vi "acq.EL.vi"(5 "Delay":u16, 6 "mode":T1, 7 "DVR":T3, 8 "error in":errorcluster, 9 "# Acq in":i32, 10 "image":refnum<queue>) -> (0 "error out":errorcluster, 2 "Image Out":T2)   [LabVIEW 2020]
uses:
  6ca06af8-5255-4aa7-8013-97f442914d80.vi
  camera/camera.lvclass
  _controls/data.ref.ctl
  _controls/data.ctl
  _controls/state.ctl
  _controls/data.vars.ctl
  _controls/flip.ctl
  <vilib>/vision/Image Controls.llb/IMAQ Image.ctl
  _controls/mode.ctl
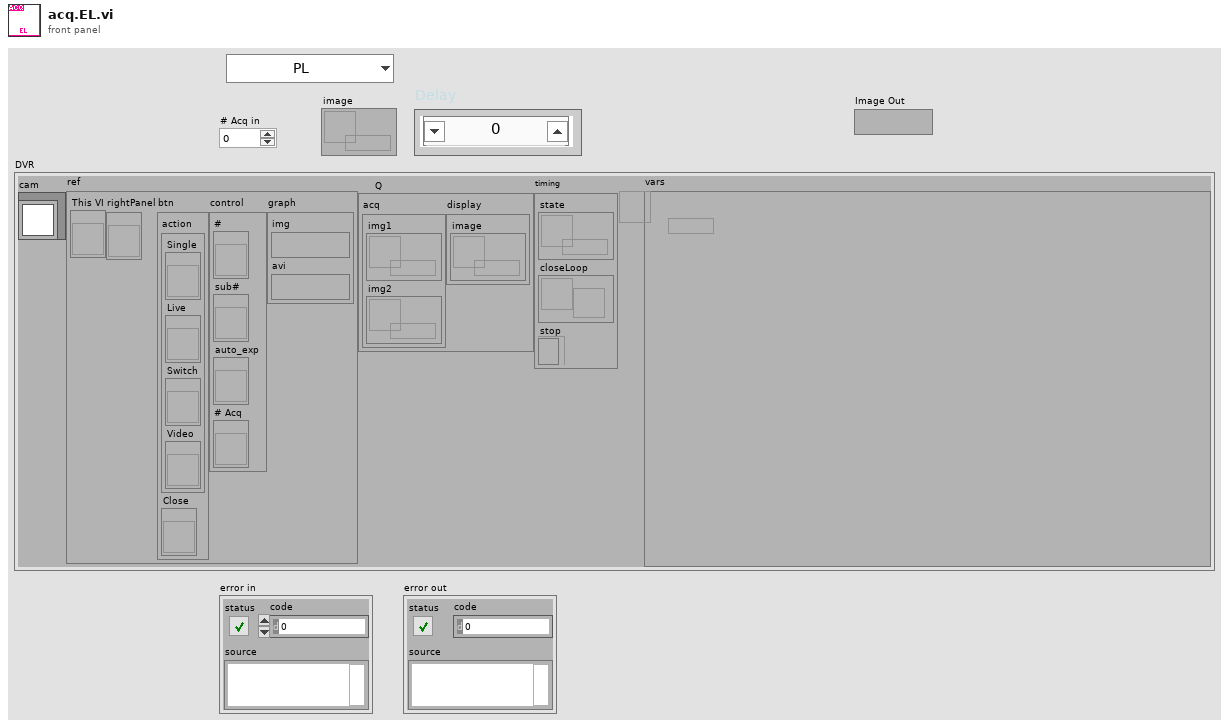
[diagram p1: front panel]
types:
  T1 = typedef "mode.ctl" = enum16{"PL", "EL"}
  T2 = typedef "IMAQ Image.ctl" = refnum<image>
  T3 = typedef "data.ctl" = cluster{"cam":refnum<class "camera.lvclass">, "ref":T4, "Q":cluster{"acq":cluster{"img1":refnum<queue>, "img2":refnum<queue>}, "display":cluster{"image":refnum<queue>}}, "timing":cluster{"state":refnum<queue>, "closeLoop":refnum<notifier>, "stop":refnum<k4>}, "vars":refnum<data-value>}
  T4 = typedef "data.ref.ctl" = cluster{"This VI":refnum<vi>, "rightPanel":refnum<vi>, "btn":cluster{"action":cluster{"Single":refnum<vi>, "Live":refnum<vi>, "Switch":refnum<vi>, "Video":refnum<vi>}, "Close":refnum<vi>}, "control":cluster{"#":refnum<vi>, "sub#":refnum<vi>, "auto_exp":refnum<vi>, "# Acq":refnum<vi>}, "graph":cluster{"img":T2, "avi":T2}}
  T5 = cluster{"img1":refnum<queue>, "img2":refnum<queue>}
  T6 = typedef "path.ctl" = cluster{"light":path, "name":string, "full":path}
  T7 = typedef "data.vars.ctl" = cluster{"save":cluster{"base_folder":cluster{"Folder":path, "tif":bool, "jpg":bool}, "module":string, "#":u32, "sub#":u8, "save.op":enum16{"Full", "Light"}, "same?":bool, "Shift":enum16{"Single", "Leapfrog"}, "jpg?":bool, "flip":T8}, "acq":cluster{"# Acq":u16, "rotate":bool, "FPS":dbl}, "calib.manual":cluster{"BG":cluster{"Image":u16[][], "enabled?":bool}, "FF":cluster{"Image":u16[][], "enabled?":bool}}}
  T8 = typedef "flip.ctl" = cluster{"x":bool, "y":bool}
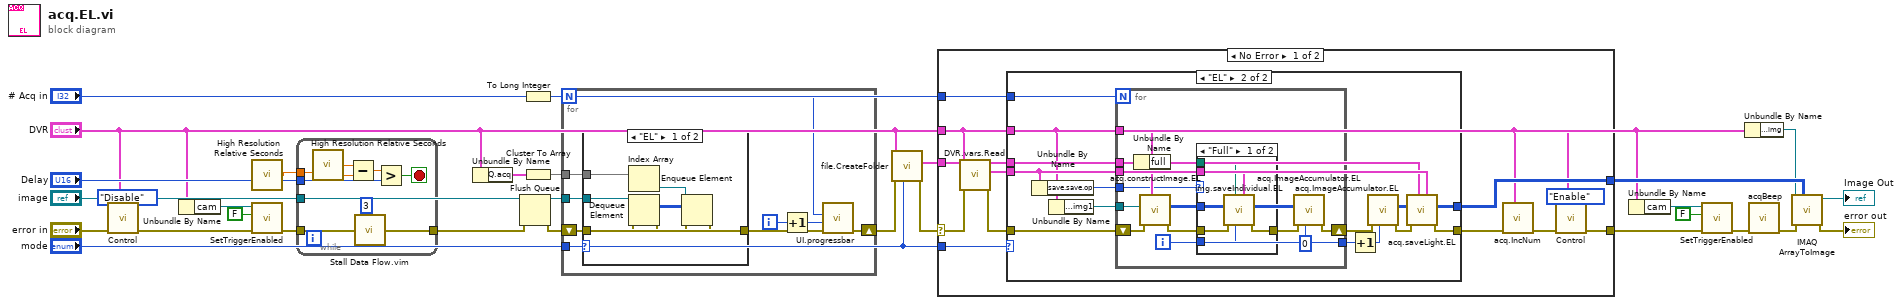
[diagram p0: block diagram]
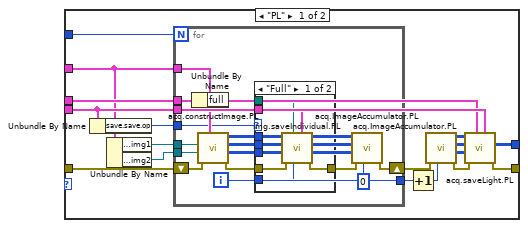
[diagram p2: hidden frame]
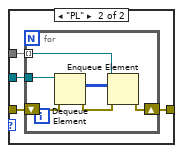
[diagram p6: hidden frame]
diagram:
  n1 = call "Control.vi"("mode"=enum16{"Enable", "Disable"}."Disable", "DVR"="DVR", "error in"="error in") -> ("error out"=w13:errorcluster)  [unwired: 8 in]
  n2 = Unbundle By Name("DVR") -> ("cam"=w14:refnum<class "camera.lvclass">)
  n3 = call <vilib>:"High Resolution Relative Seconds.vi"() -> ("relative seconds"=w18:dbl)
  n4 = call "SetTriggerEnabled.vi"("error in"=w13, "trigger"=FALSE, "camera.nit in"=w14) -> ("error out"=w12:errorcluster)  [unwired: 8 in]
  n5 = while {
    tunnel: "image" -> [_]
    tunnel: w18 -> [w36]
    tunnel: "Delay" -> [w34]
    tunnel: [w31] -> w5
    tunnel: w12 -> [w32]
    stop <- w33 stop-if-true
    n6 = call <vilib>:"High Resolution Relative Seconds.vi"() -> ("relative seconds"=w37:dbl)
    n7 = Subtract(x=w37, y=w36) -> (x-y=w35:dbl)
    n8 = call "Stall Data Flow.vim"("value in"=w32, "milliseconds to wait"=u32 3) -> ("value out"=w31:errorcluster)  [unwired: 1 out]
    n9 = Greater?(x=w35, y=w34) -> (0:w33:bool)
  }
  n10 = Unbundle By Name("DVR") -> ("Q.acq"=w23:T5)
  n11 = Flush Queue(queue="image", error in (no error)=w5) -> (queue out=w6:refnum<queue>, error out=w4:errorcluster)  [unwired: 1 out]
  n12 = To Long Integer(number="# Acq in") -> (32bit integer=w20:i32)
  n13 = Cluster To Array(cluster=w23) -> (array=w22:refnum<queue>[])
  n14 = for {
    N: w20 -> [w41]
    tunnel: w22 -> [w46]
    tunnel: w6 -> [w44]
    shift-right: [w40] -> _
    shift-left: w4 -> [w45]
    tunnel: "mode" -> [w38]
    i -> [w42]
    n15 = case shown="\"EL\"" w38 {
      tunnel: w46 -> [w53 w57]
      tunnel: w45 -> [w52 w56]
      tunnel: w44 -> [w51 w55]
      tunnel: [w50 w54] -> w43
      frame "EL" {
        n16 = Index Array(array=w53) -> (element=w47:refnum<queue>)  [unwired: 1 in]
        n17 = Dequeue Element(queue=w51, error in (no error)=w52) -> (element=w49:u16[][], error out=w48:errorcluster)  [unwired: 1 in, 2 out]
        n18 = Enqueue Element(queue=w47, element=w49, error in (no error)=w48) -> (error out=w50:errorcluster)  [unwired: 1 in, 2 out]
      }
      frame "PL" {
        n19 = for {
          tunnel: w55 -> [w63]
          tunnel: w57 -> [w62] mode=indexing
          shift-right: [w59] -> w54
          shift-left: w56 -> [w58]
          n20 = Dequeue Element(queue=w63, error in (no error)=w58) -> (element=w61:u16[][], error out=w60:errorcluster)  [unwired: 1 in, 2 out]
          n21 = Enqueue Element(queue=w62, element=w61, error in (no error)=w60) -> (error out=w59:errorcluster)  [unwired: 1 in, 2 out]
        }
      }
    }
    n22 = Increment(x=w42) -> (x+1=w39:i32)
    n23 = call "UI.progressbar.vi"("error in"=w43, "Value"=w39, "Maximum"=w41) -> ("error out"=w40:errorcluster)  [unwired: 8 in]
  }
  n24 = call "file.CreateFolder.vi"("mode"="mode", "error in"=w4, "DVR"="DVR") -> ("error out"=w29:errorcluster, "path"=w28:T6)  [unwired: 7 in]
  n25 = case shown="No Error" w29 {
    selector: w29 -> [w65 w152]
    tunnel: w20 -> [w75 _]
    tunnel: "DVR" -> [w67 _]
    tunnel: [w72 w152] -> w11
    tunnel: [w69 _] -> w27
    tunnel: w28 -> [w68 _]
    tunnel: "mode" -> [w64 _]
    frame No Error {
      n26 = call "DVR.vars.Read.vi"("error in"=w65, "DVR.state"=w67) -> ("error out"=w74:errorcluster, "vars"=w70:T7)  [unwired: 8 in]
      n27 = case shown="\"EL\"" w64 {
        tunnel: w75 -> [w92 w131]
        tunnel: w74 -> [w91 w130]
        tunnel: [w90 w129] -> w71
        tunnel: w70 -> [w89 w128]
        tunnel: [w88 w127] -> w69
        tunnel: w68 -> [w86 w125]
        tunnel: w67 -> [w79 w120]
        frame "PL" {
          n28 = Unbundle By Name(w89) -> ("save.save.op"=w87:enum16{"Full", "Light"})
          n29 = Unbundle By Name(w79) -> ("Q.acq.img1"=w78:refnum<queue>, "Q.acq.img2"=w77:refnum<queue>)
          n30 = for {
            N: w92 -> [_]
            shift-right: [w95] -> w76
            shift-left: w91 -> [w105]
            tunnel: w86 -> [w108]
            tunnel: w77 -> [w106]
            tunnel: w78 -> [w107]
            tunnel: w79 -> [w104]
            tunnel: w89 -> [w102]
            tunnel: w87 -> [w101]
            tunnel: [w94] -> w81
            i -> [w94]
            n31 = Unbundle By Name(w108) -> ("full"=w100:path)
            n32 = call "acq.constructImage.PL.vi"("DVR"=w104, "error in"=w105, "queue2 in"=w106, "queue1 in"=w107) -> ("error out"=w103:errorcluster, "Dark"=w97:u16[][], "PL"=w98:u16[][], "Bright"=w99:u16[][])  [unwired: 4 in]
            n33 = case shown="\"Full\"" w101 {
              tunnel: w100 -> [w116 _]
              tunnel: w103 -> [w115 w117]
              tunnel: w94 -> [w109 _]
              tunnel: w99 -> [w114 _]
              tunnel: w98 -> [w113 _]
              tunnel: w102 -> [w112 _]
              tunnel: w97 -> [w111 _]
              tunnel: [w110 w117] -> w96
              frame "Full" {
                n34 = call "img.saveIndividual.PL.vi"("vars"=w112, "loop"=w109, "path"=w116, "error in"=w115, "Dark"=w111, "PL"=w113, "Bright"=w114) -> ("error out"=w110:errorcluster)  [unwired: 4 in]
              }
              frame "Light" {
              }
            }
            n35 = call "acq.ImageAccumulator.PL.vi"("loop"=0, "error in"=w96, "Dark in"=w97, "PL in"=w98, "Bright in"=w99) -> ("error out"=w95:errorcluster)  [unwired: 3 in, 3 out]
          }
          n36 = Increment(x=w81) -> (x+1=w80:i32)
          n37 = call "acq.ImageAccumulator.PL.vi"("loop"=w80, "error in"=w76) -> ("error out"=w85:errorcluster, "Dark out"=w84:u16[][], "PL out"=w83:u16[][], "Bright out"=w82:u16[][])  [unwired: 6 in]
          n38 = call "acq.saveLight.PL.vi"("vars"=w89, "path"=w86, "error in"=w85, "Dark"=w84, "PL"=w83, "Bright"=w82) -> ("error out"=w90:errorcluster, "PL"=w88:u16[][])  [unwired: 3 in, 1 out]
        }
        frame "EL" {
          n39 = Unbundle By Name(w128) -> ("save.save.op"=w126:enum16{"Full", "Light"})
          n40 = Unbundle By Name(w120) -> ("Q.acq.img1"=w119:refnum<queue>)
          n41 = for {
            N: w131 -> [_]
            shift-right: [w134] -> w118
            shift-left: w130 -> [w142]
            tunnel: w125 -> [w144]
            tunnel: w119 -> [w143]
            tunnel: w120 -> [w141]
            tunnel: w128 -> [w139]
            tunnel: w126 -> [w138]
            tunnel: [w133] -> w122
            i -> [w133]
            n42 = Unbundle By Name(w144) -> ("full"=w137:path)
            n43 = call "acq.constructImage.EL.vi"("DVR"=w141, "error in"=w142, "queue1 in"=w143) -> ("error out"=w140:errorcluster, "EL"=w136:u16[][])  [unwired: 7 in]
            n44 = case shown="\"Full\"" w138 {
              tunnel: w137 -> [w150 _]
              tunnel: w140 -> [w149 w151]
              tunnel: w133 -> [w145 _]
              tunnel: w136 -> [w148 _]
              tunnel: w139 -> [w147 _]
              tunnel: [w146 w151] -> w135
              frame "Full" {
                n45 = call "img.saveIndividual.EL.vi"("vars"=w147, "loop"=w145, "path"=w150, "error in"=w149, "EL"=w148) -> ("error out"=w146:errorcluster)  [unwired: 6 in]
              }
              frame "Light" {
              }
            }
            n46 = call "acq.ImageAccumulator.EL.vi"("loop"=0, "error in"=w135, "EL in"=w136) -> ("error out"=w134:errorcluster)  [unwired: 7 in, 1 out]
          }
          n47 = Increment(x=w122) -> (x+1=w121:i32)
          n48 = call "acq.ImageAccumulator.EL.vi"("loop"=w121, "error in"=w118) -> ("error out"=w124:errorcluster, "EL out"=w123:u16[][])  [unwired: 8 in]
          n49 = call "acq.saveLight.EL.vi"("vars"=w128, "path"=w125, "error in"=w124, "EL"=w123) -> ("error out"=w129:errorcluster, "EL"=w127:u16[][])  [unwired: 6 in]
        }
      }
      n50 = call "acq.IncNum.vi"("DVR in"=w67, "error in"=w71) -> ("error out"=w66:errorcluster)  [unwired: 9 in]
      n51 = call "Control.vi"("mode"=enum16{"Enable", "Disable"}."Enable", "DVR"=w67, "error in"=w66) -> ("error out"=w72:errorcluster)  [unwired: 8 in]
    }
    frame Error {
    }
  }
  n52 = Unbundle By Name("DVR") -> ("cam"=w9:refnum<class "camera.lvclass">)
  n53 = call "SetTriggerEnabled.vi"("error in"=w11, "trigger"=FALSE, "camera.nit in"=w9) -> ("error out"=w8:errorcluster)  [unwired: 8 in]
  n54 = Unbundle By Name("DVR") -> ("ref.graph.img"=w24:T2)
  n55 = call "acqBeep.vi"("error in"=w8) -> ("error out"=w7:errorcluster)  [unwired: 10 in]
  n56 = call "IMAQ ArrayToImage"("Image Pixels (U16)"=w27, "error in (no error)"=w7, "Image"=w24) -> ("error out"=→"error out":errorcluster, "Image Out"=→"Image Out":T2)  [unwired: 7 in]
